vi "Pixel2mm.vi"(11 "Numeric in":sgl) -> (3 "Numeric out":dbl)   [LabVIEW 2019, in "Algorithm.lvclass"]
doc: "Applies the calibration information and converts the distance in pixels to mm"
uses:
  FrameworkOverrides/Algorithm.lvclass
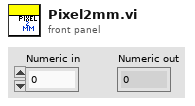
[diagram p1: front panel]
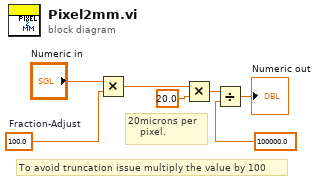
[diagram p0: block diagram]
diagram:
  w2 = 100.0  # Fraction-Adjust
  # "20microns per \n    pixel."
  # "To avoid truncation issue multiply the value by 100"
  n1 = Multiply(x="Numeric in", y=w2) -> (x*y=w4:dbl)
  n2 = Multiply(x=w4, y=20.0) -> (x*y=w5:dbl)
  n3 = Divide(x=w5, y=100000.0) -> (x/y=→"Numeric out":dbl)
